vi "Y1subvi.vi"(4 "MAXIMUM":ext format="%.9f", 6 "MINIMUM":ext format="%.9f", 8 "error in (no error)":errorcluster, 9 "LIN or LOG axis":string, 10 "Variable name":string, 11 "VISA In":refnum<visa-resource-name>) -> (0 "error out":errorcluster, 3 "VISA Out":refnum<visa-resource-name>)   [LabVIEW 2012]
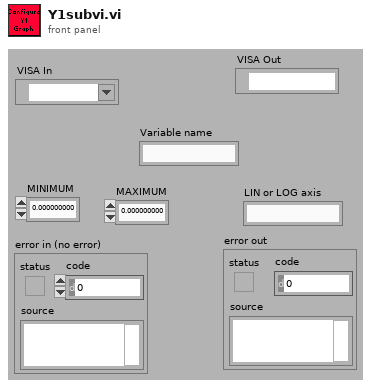
[diagram p1: front panel]
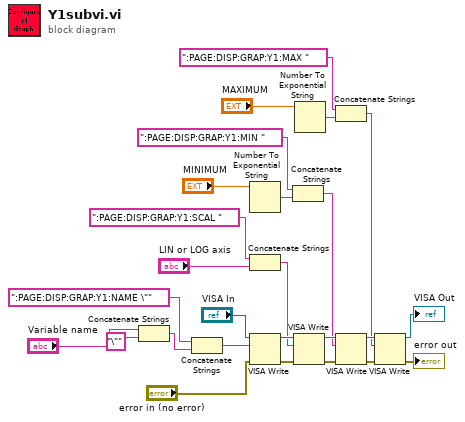
[diagram p0: block diagram]
diagram:
  n1 = Concatenate Strings("Variable name", "\"" ("string")) -> (w24:string)
  n2 = Concatenate Strings(":PAGE:DISP:GRAP:Y1:NAME \"" ("write buffer"), w24) -> (w21:string)
  n3 = Number To Exponential String(number="MINIMUM") -> (E-format string=w9:string)  [unwired: 3 in]
  n4 = Concatenate Strings(":PAGE:DISP:GRAP:Y1:SCAL " ("write buffer"), "LIN or LOG axis") -> (w12:string)
  n5 = VISA Write(VISA resource name="VISA In", write buffer=w21, error in (no error)="error in (no error)") -> (VISA resource name out=w20:refnum<visa-resource-name>, error out=w17:errorcluster)  [unwired: 1 out]
  n6 = Concatenate Strings(":PAGE:DISP:GRAP:Y1:MIN " ("write buffer"), w9) -> (w8:string)
  n7 = VISA Write(VISA resource name=w20, write buffer=w12, error in (no error)=w17) -> (VISA resource name out=w19:refnum<visa-resource-name>, error out=w16:errorcluster)  [unwired: 1 out]
  n8 = Number To Exponential String(number="MAXIMUM") -> (E-format string=w7:string)  [unwired: 3 in]
  n9 = Concatenate Strings(":PAGE:DISP:GRAP:Y1:MAX " ("write buffer"), w7) -> (w4:string)
  n10 = VISA Write(VISA resource name=w19, write buffer=w8, error in (no error)=w16) -> (VISA resource name out=w18:refnum<visa-resource-name>, error out=w15:errorcluster)  [unwired: 1 out]
  n11 = VISA Write(VISA resource name=w18, write buffer=w4, error in (no error)=w15) -> (VISA resource name out=→"VISA Out":refnum<visa-resource-name>, error out=→"error out":errorcluster)  [unwired: 1 out]
